vi "getKeyOrIndex.vi"(8 "error in (no error)":errorcluster, 11 "input string":string) -> (0 "error out":errorcluster, 1 "value":string, 2 "key":string, 3 "index":i32, 5 "keygiven?":bool)   [LabVIEW 2015, in "Zen Analytics.lvclass"]
uses:
  Zen Analytics.lvclass
  <vilib>/regexp/Match Regular Expression.xnode
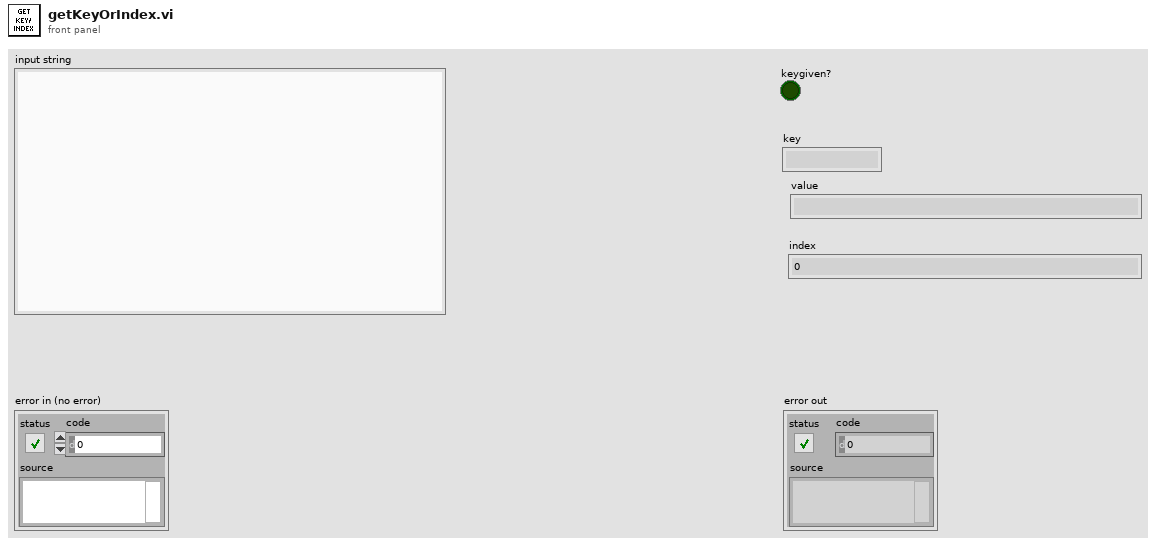
[diagram p1: front panel]
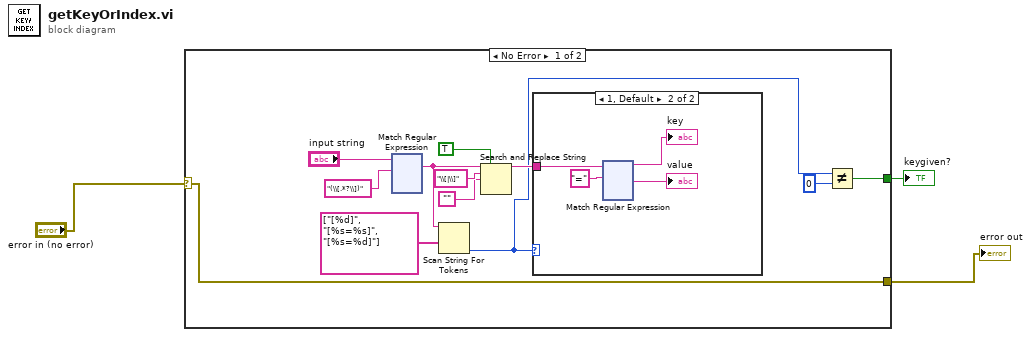
[diagram p0: block diagram]
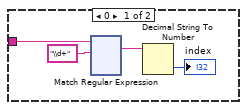
[diagram p2: hidden frame]
diagram:
  n1 = case shown="No Error" "error in (no error)" {
    selector: "error in (no error)" -> [w7 w366]
    tunnel: [w7 w366] -> w2
    tunnel: [w4 _] -> w1
    frame No Error {
      n2 = xnode "Match Regular Expression"("input string"="input string", "regular expression"="(\\[.*?\\])") -> ("whole match"=w12:string)  [unwired: 4 in, 4 out]
      n3 = Scan String For Tokens(7:string[] ["[%d]", "[%s=%s]", "[%s=%d]"] ("operators (none)"), 9:w12) -> (0:w6:i32)  [unwired: 4 in, 3 out]
      n4 = Search and Replace String(replace all?=TRUE ("replace all? (F)"), input string=w12, search string="\\[|\\]", replace string="") -> (result string=w9:string)  [unwired: 4 in, 3 out]
      n5 = case shown="1, Default" w6 {
        tunnel: w9 -> [w19 w137]
        frame 0 {
          n6 = xnode "Match Regular Expression"("input string"=w19, "regular expression"="\\d+") -> ("whole match"=w17:string)  [unwired: 4 in, 4 out]
          n7 = Decimal String To Number(string=w17) -> (number=→"index":i32)  [unwired: 2 in, 1 out]
        }
        frame 1, Default {
          n8 = xnode "Match Regular Expression"("input string"=w137, "regular expression"="=") -> ("before match"=→"key":string, "after match"=→"value":string)  [unwired: 4 in, 3 out]
        }
      }
      n9 = Not Equal?(x=w6, y=0) -> (x != y?=w4:bool)
    }
    frame Error {
    }
  }
  "error out" <- w2
  "keygiven?" <- w1
